vi "HTTP.Send.vi"(8 "error in (no error)":errorcluster, 9 "body":string, 10 "Status LIne":string, 11 "Connection.WS in":refnum<class "Connection.WS.lvclass">) -> (0 "error out":errorcluster, 3 "Connection.WS out":refnum<class "Connection.WS.lvclass">)   [LabVIEW 2013, in "Connection.WS_GOSPL.lvlib" / "Connection.WS.lvclass"]
uses:
  Connection.WS.lvclass
  Header Fields -- combo.ctl
  Connection/Connection.lvclass/Connection.ctl
  Connection.WS.lvclass/Connection.WS.ctl
  Connection/Connection.lvclass
  Connection.TCP/Connection.TCP.lvclass
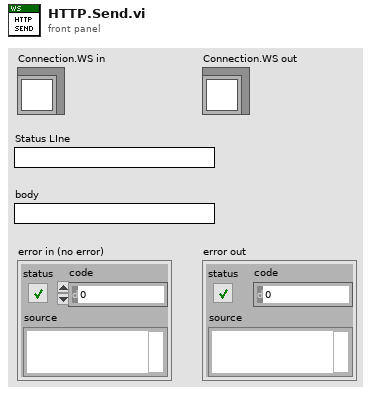
[diagram p1: front panel]
types:
  T1 = typedef "Connection.WS_GOSPL.lvlib/Connection.WS.lvclass/Header Fields -- combo.ctl" = string
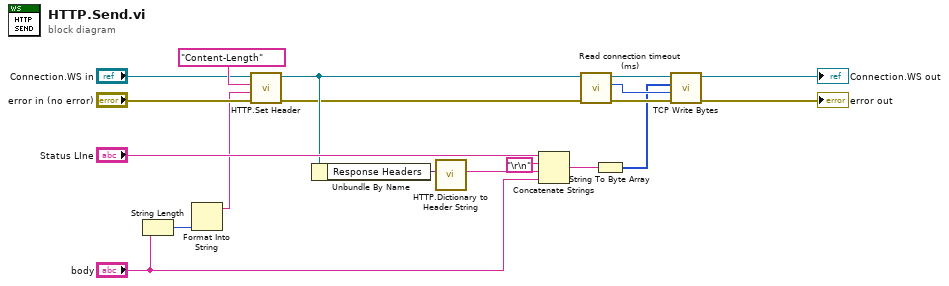
[diagram p0: block diagram]
diagram:
  n1 = String Length(string="body") -> (length=w2:i32)
  n2 = Format Into String(w2) -> (resulting string=w1:string)  [unwired: 3 in, 1 out]
  n3 = call "HTTP.Set Header.vi"("error in (no error)"="error in (no error)", "Value"=w1, "Header Name"=T1 "Content-Length", "Connection.WS in"="Connection.WS in") -> ("error out"=w3:errorcluster, "Connection.WS out"=w5:refnum<class "Connection.WS.lvclass">)  [unwired: 6 in]
  n4 = Unbundle By Name(w5) -> ("Response Headers"=w19:variant)
  n5 = call "HTTP.Dictionary to Header String.vi"("Dictionary"=w19) -> ("HTTP Header"=w9:string)  [unwired: 10 in]
  n6 = Concatenate Strings("Status LIne", "\r\n", w9, "body") -> (w11:string)
  n7 = call "Read connection timeout (ms).vi"("error in (no error)"=w3, "Connection in"=w5) -> ("error out"=w14:errorcluster, "connection timeout (ms)"=w13:i32, "Connection out"=w15:refnum<class "Connection.WS.lvclass">)  [unwired: 7 in]
  n8 = String To Byte Array(string=w11) -> (unsigned byte array=w12:u8[])
  n9 = call "TCP Write Bytes.vi"("error in (no error)"=w14, "timeout ms (2000)"=w13, "Bytes"=w12, "Connection.TCP"=w15) -> ("error out"=→"error out":errorcluster, "Connection.TCP"=→"Connection.WS out":refnum<class "Connection.WS.lvclass">)  [unwired: 6 in]
